vi "Call (Async).vi"(0 "WAMP Client in":refnum<class "WAMP Client.lvclass">, 5 "error in (no error)":errorcluster, 7 "Topic URI":string, 9 "Arguments":variant[](array[variant]), 11 "ArgumentsKw":string) -> (4 "WAMP Client out":refnum<class "WAMP Client.lvclass">, 6 "error out":errorcluster, 15 "user event out":refnum<user-event>)   [LabVIEW 2020, in "WAMP Client.lvclass"]
uses:
  <userlib>/lvwamp/WAMP Client/WAMP Client.lvclass
  <userlib>/lvwamp/WAMP Client/TypeDef/RESULT Payload.ctl
  <userlib>/lvwamp/WAMP Client/TypeDef/WAMP Error Payload.ctl
  <userlib>/lvwamp/WAMP Client/TypeDef/Internal Message Type.ctl
  <userlib>/lvwamp/WAMP Client/TypeDef/CALL Request Data.ctl
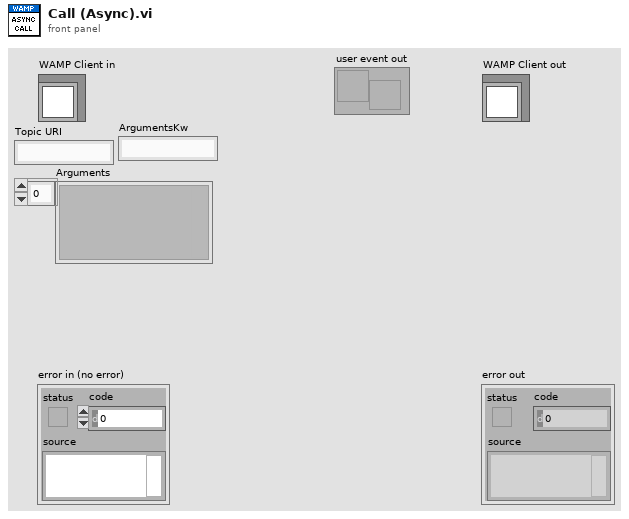
[diagram p1: front panel]
types:
  T1 = typedef "WAMP Client.lvclass/RESULT Payload.ctl" = cluster{"Arguments Payload":string[], "ArgumentKw Payload":string, "Topic":string, "Success?":bool, "WAMP Error":T2}
  T2 = typedef "WAMP Client.lvclass/WAMP Error Payload.ctl" = cluster{"Arguments Payload":string[], "ArgumentKw Payload":string, "Error URI":string, "Error?":bool}
  T3 = typedef "WAMP Client.lvclass/CALL Request Data.ctl" = cluster{"Topic URI":string, "Arguments":variant[], "ArgumentsKw":string, "Result Received":refnum<user-event>}
  T4 = typedef "WAMP Client.lvclass/Internal Message Type.ctl" = enum16{"Subscribe", "Handle Subscribed", "Handle Event", "Unsubscribe", "Handle Unsubscribed", "Publish", "Handled Published", "Goodbye", "Handle Goodbye", "Call", "Handle Result"}
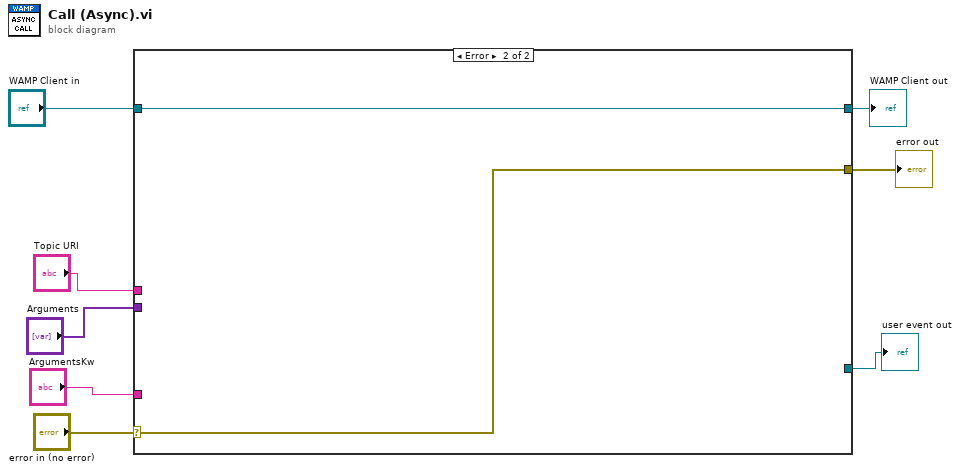
[diagram p0: block diagram]
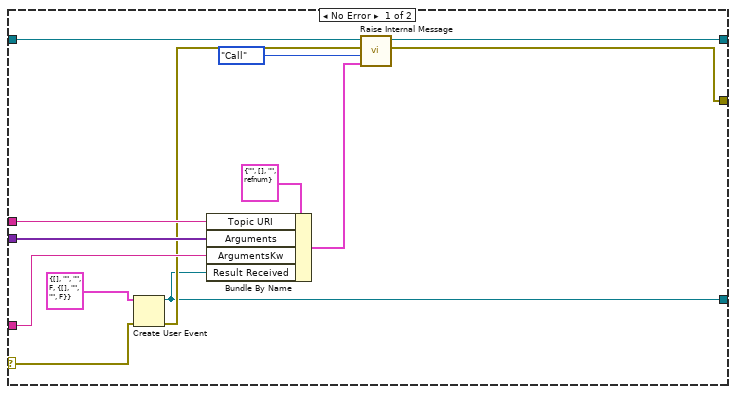
[diagram p2: hidden frame]
diagram:
  n1 = case shown="Error" "error in (no error)" {
    selector: "error in (no error)" -> [w11 w23]
    tunnel: [w18 w23] -> w7
    tunnel: [w20 w22] -> w5
    tunnel: "WAMP Client in" -> [w21 w22]
    tunnel: "Topic URI" -> [w16 _]
    tunnel: "Arguments" -> [w15 _]
    tunnel: "ArgumentsKw" -> [w14 _]
    tunnel: [w9 _] -> w1
    frame No Error {
      n2 = Create User Event(user event datatype=T1 {"Arguments Payload"=[], "ArgumentKw Payload"="", "Topic"="", "Success?"=FALSE, "WAMP Error"={"Arguments Payload"=[], "ArgumentKw Payload"="", "Error URI"="", "Error?"=FALSE}} ("RESULT Payload"), error in=w11) -> (user event=w9:refnum<user-event>, error out=w10:errorcluster)
      n3 = Bundle By Name(cluster=T3 {"Topic URI"="", "Arguments"=[], "ArgumentsKw"="", "Result Received"=refnum} ("Call Request"), "Topic URI"=w16, "Arguments"=w15, "ArgumentsKw"=w14, "Result Received"=w9) -> (w13:T3)
      n4 = call-dynamic "Raise Internal Message.vi"("Variant"=w13, "Internal Message Type"=Internal_Message_Type."Call", "error in (no error)"=w10, "WAMP Client in"=w21) -> ("error out"=w18:errorcluster, "WAMP Client out"=w20:refnum<class "WAMP Client.lvclass">)  [unwired: 6 in]
    }
    frame Error {
    }
  }
  "error out" <- w7
  "WAMP Client out" <- w5
  "user event out" <- w1
